vi "Event.vi"() -> ()   [LabVIEW 2018]
panel:
  out "불리언":bool=TRUE
  out "시간":u32
  in  "정지":bool
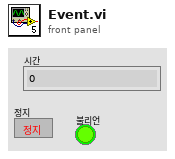
[diagram p1: front panel]
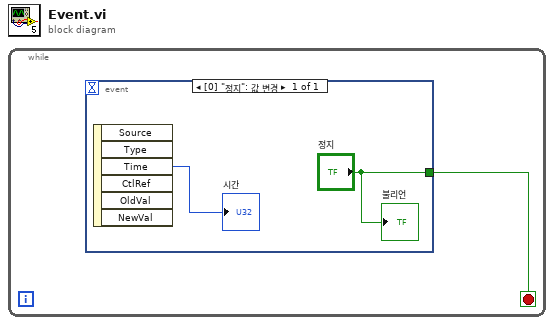
[diagram p0: block diagram]
diagram:
  n1 = while {
    stop <- w1 stop-if-true
    n2 = event shown="[0] \"정지\": 값 변경" {
      selector: _ -> [_]
      dyn-events: _ -> [_]
      timeout: _ -> [_]
      tunnel: ["정지"] -> w1
      event "정지": Value Change {
        n3 = event-data() -> ("Time"=→"시간":u32)  [unwired: 1 in, 5 out]
        "불리언" <- "정지"
      }
    }
  }
